vi "RegisteredMsgUpdate.vi"(8 "error in (no error)":errorcluster, 10 "Msgs":refnum<class "MailBoxMessage.lvclass">[](array[class]), 11 "Test-Client in":refnum<class "Test-Client.lvclass">) -> (0 "error out":errorcluster, 3 "Test-Client out":refnum<class "Test-Client.lvclass">)   [LabVIEW 2020, in "Test-Client.lvlib" / "Test-Client.lvclass"]
uses:
  Test-Client.lvclass
  MailboxManager/MailBoxMessage/MailBoxMessage.lvclass
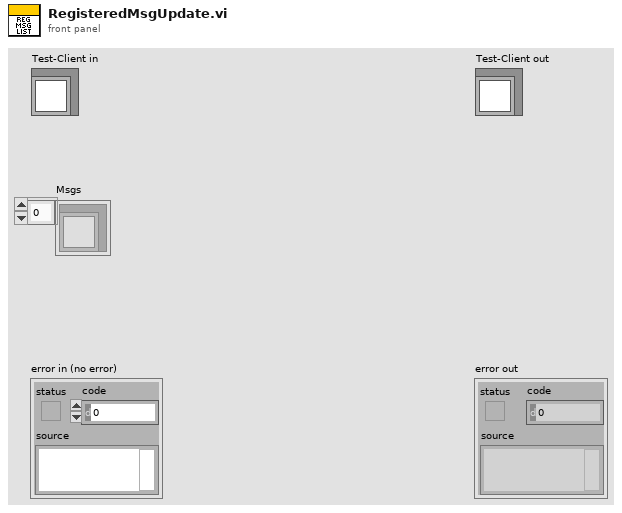
[diagram p1: front panel]
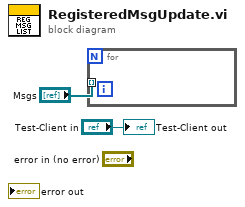
[diagram p0: block diagram]
diagram:
  n1 = for {
    tunnel: "Msgs" -> [_] mode=indexing
  }
  "Test-Client out" <- "Test-Client in"
